vi "Get Plot Properties.vi"(8 "error in (no error)":errorcluster, 11 "Scale Refnum":refnum<vi>) -> (0 "error out":errorcluster, 3 "Array":T1[](array[typedef]))   [LabVIEW 2020]
uses:
  Plot Properties.ctl
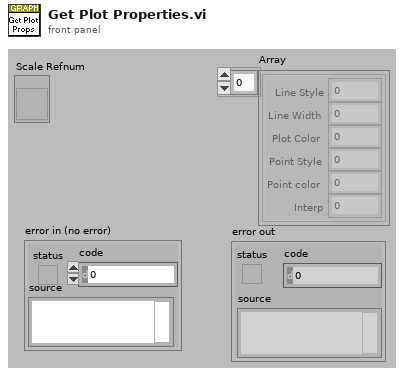
[diagram p1: front panel]
types:
  T1 = typedef "Plot Properties.ctl" = cluster{"Line Style":u8, "Line Width":u8, "Plot Color":u32, "Point Style":u8, "Point color":u32, "Interp":u8}
  T2 = cluster{"Plot.Line Style":u8, "Plot.Line Width":u8, "Plot.Plot Color":u32, "Plot.Point Style":u8, "Plot.Fill/Pt. Color":u32, "Plot.Plot Interpolation":u8}
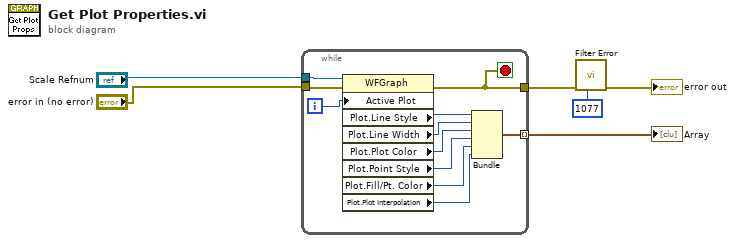
[diagram p0: block diagram]
diagram:
  n1 = while {
    tunnel: "Scale Refnum" -> [w17]
    tunnel: "error in (no error)" -> [w16]
    tunnel: [w7] -> w6
    tunnel: [w10] -> w5 mode=indexing
    i -> [w15]
    stop <- w7 stop-if-true
    n2 = property class="WFGraph"(reference=w17, error in=w16, "Active Plot"=w15) -> (error out=w7:errorcluster, "Plot.Line Style"=w14:u8, "Plot.Line Width"=w13:u8, "Plot.Plot Color"=w12:u32, "Plot.Point Style"=w11:u8, "Plot.Fill/Pt. Color"=w9:u32, "Plot.Plot Interpolation"=w8:u8)  [unwired: 1 out]
    n3 = Bundle("Plot.Line Style"=w14, "Plot.Line Width"=w13, "Plot.Plot Color"=w12, "Plot.Point Style"=w11, "Plot.Fill/Pt. Color"=w9, "Plot.Plot Interpolation"=w8) -> (w10:T2)  [unwired: 1 in]
  }
  "Array" <- w5
  n4 = call "Filter Error.vi"("error in (no error)"=w6, "code to ignore"=1077) -> ("error out"=→"error out":errorcluster)  [unwired: 9 in]
